vi "Get Cascaded Coefficients of IIR Filter.vi"() -> ()   [LabVIEW 2023]
doc: "Demonstrates how to use the DFD Get Cascaded Coef VI to convert a filter that you designed with the Digital Filter Design VIs to an infinite impulse response (IIR) filter cluster that you can use with the Filters VIs in the LabVIEW Full or Professional Development System. This example also demonstrates that the filtering results are the same when you process a signal using either the original filter or the converted filter cluster.\n\nComplete the following steps to use this VI.\n1) Run the VI.\n2) Observe the Filtered Signals graph.\n3) Observe the Forward Coefficients and Reverse Coefficients arrays from the Digital Filter Design (DFD) Toolkit and from LabVIEW.\n4) Examine the block diagram to learn how to use the Utilities VIs."
uses:
  <vilib>/addons/Digital Filter Design/Process.llb/DFD Filtering (Array).vi
  <vilib>/Analysis/baseanly.llb/IIR Cascade Filter (DBL).vi
  <vilib>/addons/Digital Filter Design/NI_DigFilterLicensed.lvlib
  <vilib>/Analysis/NI_AALBase.lvlib
panel:
  out "Reverse Coefficients from DFD":dbl[](array[numeric])
  out "Forward Coefficients from DFD":dbl[](array[numeric])
  out "Forward Coefficients from LabVIEW":dbl[](array[numeric])
  out "Reverse Coefficients from LabVIEW":dbl[](array[numeric])
  out "Filtered Signals":dbl[][](graph)
  # "Select Help>>Show Context Help and move the cursor over the VI icon for more information."
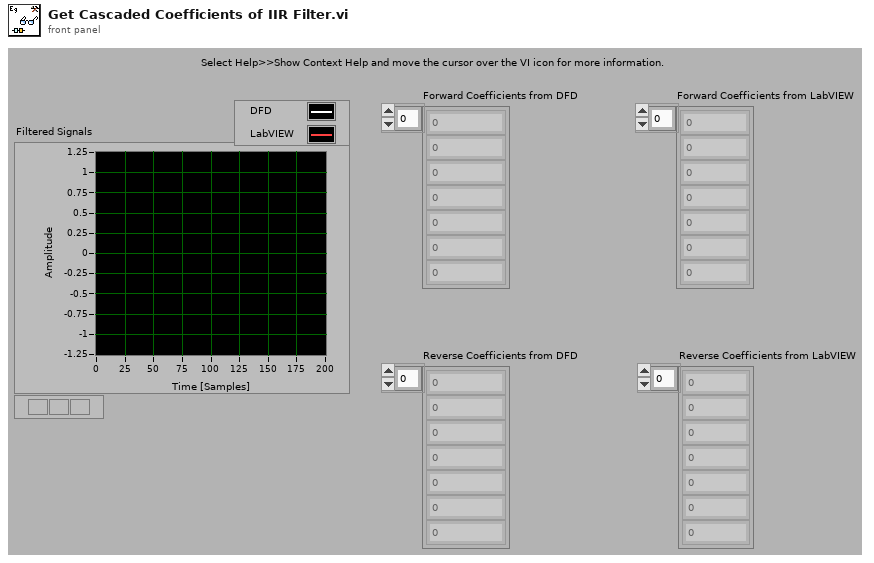
[diagram p1: front panel]
types:
  T1 = typedef "NI_DigFilterLicensed.lvlib/DFD Filter Obj.ctl" = cluster{"mSRate_Fs":dbl, "mSRate_Version":string, "mSRate_Comments":string, "mSRate_OrgCoef":T2, "mSRate_CurCoef":T2, "mSRate_Quantized?":bool, "mSRate_QCoef":T2, "mSRate_QSettings":T4[], "mSRate_Order":i32, "mSRate_Scaling":cluster{"mSRate_ScaleByPowerOf2?":bool, "mSRate_ScaleType":T6}}
  T2 = typedef "NI_DigFilterLicensed.lvlib/DFD Filter Coef.ctl" = cluster{"type":T3, "gain":dbl, "coef a (k)":dbl[], "coef b (v)":dbl[]}
  T3 = typedef "NI_DigFilterLicensed.lvlib/DFD Filter Structure Type Selector.ctl" = enum16{"Undefined", "FIR Direct Form", "FIR Direct Form Transposed", "FIR Symmetric", "FIR Antisymmetric", "IIR Direct Form I", "IIR Direct Form I Transposed", "IIR Direct Form II", "IIR Direct Form II Transposed", "IIR Cascaded Second Order Sections Form I", "IIR Cascaded Second Order Sections Form I Transposed", "IIR Cascaded Second Order Sections Form II", "IIR Cascaded Second Order Sections Form II Transposed", "Lattice Allpass (basic sections)", "Lattice Allpass (one multiplier sections)", "Lattice Allpass (normalized sections)", "Lattice AR (basic sections)", "Lattice AR (one multiplier sections)", "Lattice AR (normalized sections)", "Lattice MA (minimum phase)", "Lattice MA (maximum phase)", "Lattice ARMA (basic sections)", "Lattice ARMA (one multiplier sections)", "Lattice ARMA (normalized sections)"}
  T4 = typedef "NI_DigFilterLicensed.lvlib/dfd_Internal Quantization Settings.ctl" = cluster{"source":T5, "wl":i16, "iwl":i16, "overflow mode":enum16{"Saturation", "Wrap"}, "rounding mode":enum16{"Nearest", "Truncation"}, "signed?":bool}
  T5 = typedef "NI_DigFilterLicensed.lvlib/dfd_Internal Quantization Srcs.ctl" = u16
  T6 = typedef "NI_DigFilterLicensed.lvlib/DFD Coef Norm Type.ctl" = enum16{"No Norm", "Time Domain 1-Norm", "Time Domain 2-Norm", "Time Domain Inf-Norm"}
  T7 = cluster{"filter structure":enum32{"IIR 2nd Order", "IIR 4th Order"}, "Reverse Coefficients":dbl[], "Forward Coefficients":dbl[]}
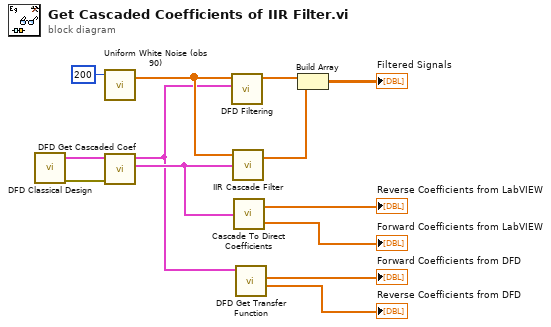
[diagram p0: block diagram]
diagram:
  n1 = call <vilib>:"DFD Classical Design.vi"() -> ("error out"=w12:errorcluster, "filter out"=w13:T1)  [unwired: 6 in, 4 out]
  n2 = call <vilib>:"Uniform White Noise (obs 90).vi"("samples"=200) -> ("uniform white noise"=w9:dbl[])  [unwired: 2 in, 1 out]
  n3 = call <vilib>:"DFD Get Cascaded Coef.vi"("error in (no error)"=w12, "filter in"=w13) -> ("IIR Filter Cluster"=w11:T7, "filter out"=w5:T1)  [unwired: 8 out]
  n4 = call-poly <vilib>:"DFD Filtering.vi"("filter"=w5, "signal in"=w9) -> ("signal out"=w8:dbl[])  [unwired: 2 in, 7 out]
  n5 = call-poly <vilib>:"IIR Cascade Filter.vi"("IIR Filter Cluster"=w11, "X"=w9) -> ("Filtered X"=w7:dbl[])  [unwired: 1 in, 1 out]
  n6 = call <vilib>:"Cascade To Direct Coefficients.vi"("IIR Filter Cluster"=w11) -> ("Reverse Coefficients"=→"Reverse Coefficients from LabVIEW":dbl[], "Forward Coefficients"=→"Forward Coefficients from LabVIEW":dbl[])
  n7 = call <vilib>:"DFD Get Transfer Function.vi"("filter in"=w5) -> ("denominator"=→"Reverse Coefficients from DFD":dbl[], "numerator"=→"Forward Coefficients from DFD":dbl[])  [unwired: 1 in, 8 out]
  n8 = Build Array(w8, w7) -> (→"Filtered Signals":dbl[][])
